vi "Read _LangData.vi"(8 "error in (no error)":errorcluster, 11 "UI View in":refnum<class "UI View.lvclass">) -> (0 "error out":errorcluster, 2 "*LangData":refnum<data-value>, 3 "UI View out":refnum<class "UI View.lvclass">)   [LabVIEW 2013, in "SET Project Editor.lvlib" / "UI View.lvclass"]
uses:
  UI View.lvclass
  SET Project Data/Project Data Class/Project Data.lvclass
  UI View.lvclass/UI View.ctl
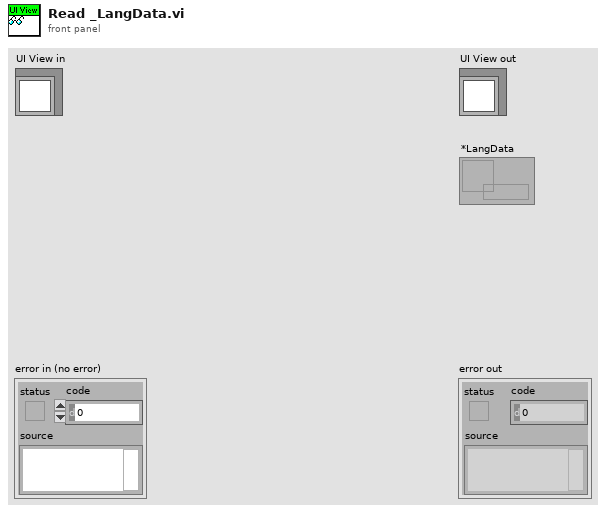
[diagram p1: front panel]
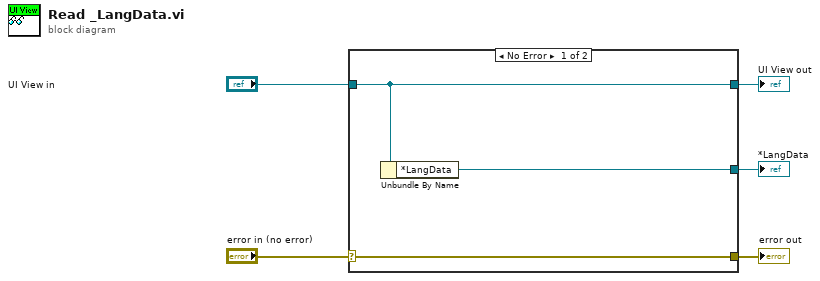
[diagram p0: block diagram]
diagram:
  n1 = case shown="No Error" "error in (no error)" {
    selector: "error in (no error)" -> [w8 w9]
    tunnel: [w8 w9] -> w4
    tunnel: [w7 w10] -> w2
    tunnel: "UI View in" -> [w7 w10]
    tunnel: [w6 _] -> w1
    frame No Error {
      n2 = Unbundle By Name(w7) -> ("*LangData"=w6:refnum<data-value>)
    }
    frame Error {
    }
  }
  "error out" <- w4
  "UI View out" <- w2
  "*LangData" <- w1
